vi "Power ON-Single.vi"(8 "error in":errorcluster, 11 "Power ON single":T1={"Voltage/current level"=0.0, "Voltage/current limit"=0.0, "Sense"=1009, "Resource name"="", "Output function"=1006} {"Output function" items=["DC Voltage"=1006, "DC Current"=1007, "Pulse Voltage"=1049, "Pulse Current"=1050]; "Sense" items=["Local"=1008, "Remote"=1009]}) -> (0 "error out":errorcluster, 3 "Status":string)   [LabVIEW 2021]
doc: "This VI will configure the source device to DC Current or DC Voltage mode to ower on the DUT for single channel configuration."
uses:
  controls/Power ON-Single.ctl
  <instrlib>/niDCPower/nidcpower.llb/niDCPower Source Mode.ctl
  <instrlib>/niDCPower/nidcpower.llb/niDCPower Wait For Event - Event.ctl
  <instrlib>/niDCPower/nidcpower.llb/niDCPower Get Channel Name From String.vi
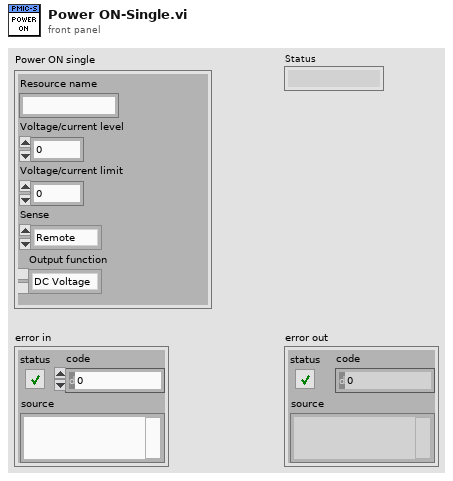
[diagram p1: front panel]
types:
  T1 = typedef "Power ON-Single.ctl" = cluster{"Voltage/current level":dbl, "Voltage/current limit":dbl, "Sense":i32, "Resource name":string, "Output function":i32}
  T2 = typedef "niDCPower Wait For Event - Event.ctl" = i32
  T3 = typedef "niDCPower Source Mode.ctl" = i32
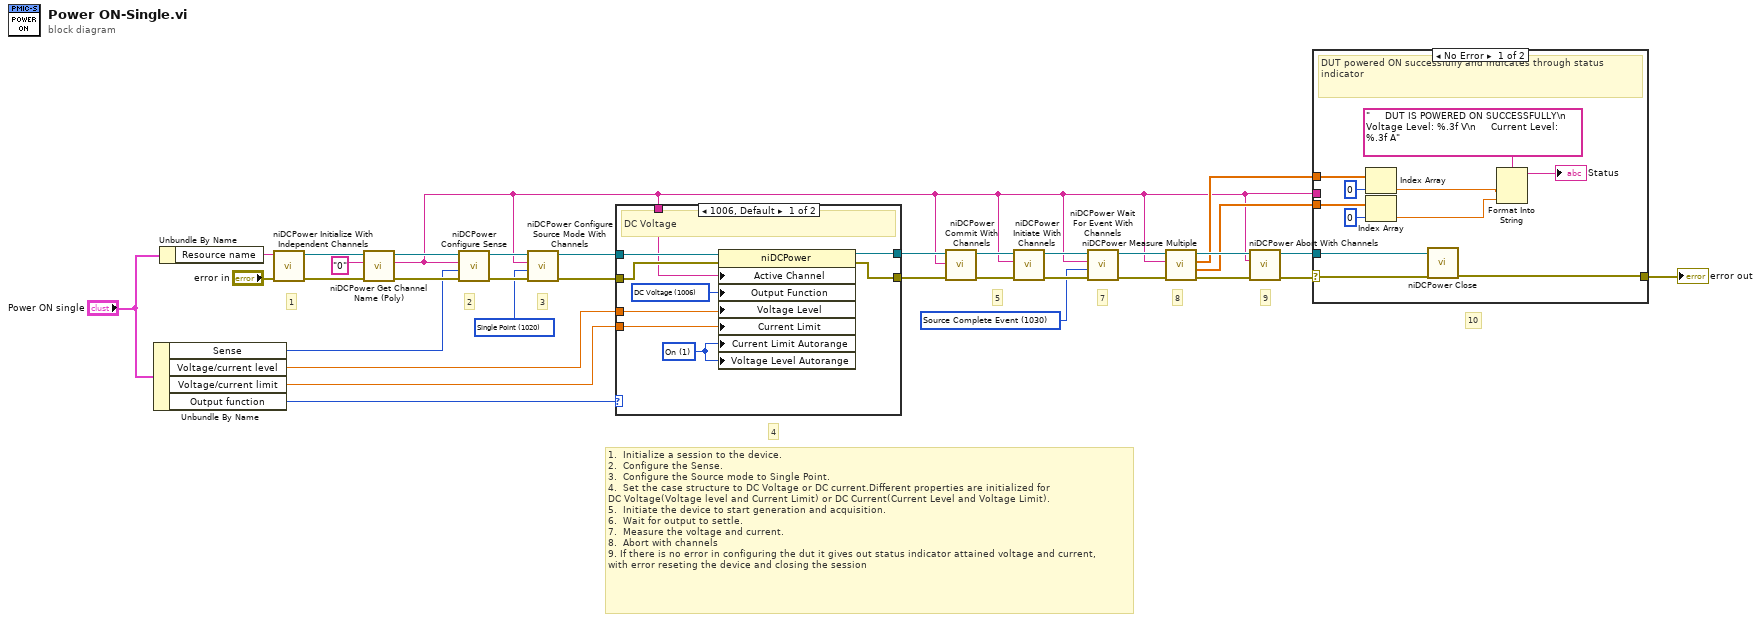
[diagram p0: block diagram]
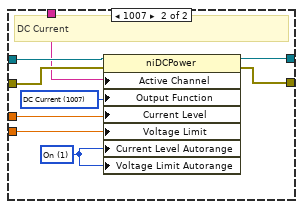
[diagram p2: hidden frame]
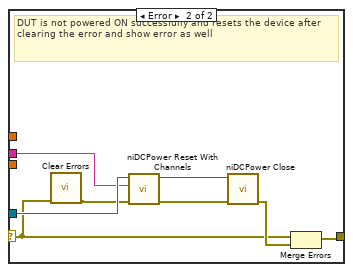
[diagram p3: hidden frame]
diagram:
  w22 = T2 1030 items=["Source Complete Event"=1030, "Measure Complete Event"=1031, "Sequence Iteration Complete Event"=1032, "Sequence Engine Done Event"=1033, "Pulse Complete Event"=1051, "Ready For Pulse Trigger Event"=1052] ("event")
  w27 = T3 1020 items=["Single Point"=1020, "Sequence"=1021] ("source mode")
  # "10"
  # "9"
  # "8"
  # "7"
  # "5"
  # "4"
  # "3"
  # "2"
  # "1"
  # "1.  Initialize a session to the device.\n2.  Configure the Sense.\n3.  Configure the Source mode to Single Point.\n4.  Set the case structure to DC Voltage or DC current.Different properties are initialized for \nDC Voltage(Voltage level and Current Limit) or DC Current(Current Level and Voltage Limit). \n5.  Initiate the device to start generation and acquisition.\n6.  Wait for output to settle.\n7.  Measure the voltage and current.\n8.  Abort with channels\n9. If there is no error in configuring the dut it gives out status indicator attained voltage and current,\nwith error reseting the device and closing the session"
  n1 = Unbundle By Name("Power ON single") -> ("Sense"=w1:i32, "Voltage/current level"=w7:dbl, "Voltage/current limit"=w6:dbl, "Output function"=w5:i32)
  n2 = Unbundle By Name("Power ON single") -> ("Resource name"=w13:string)
  n3 = call <instrlib>:"niDCPower Initialize With Independent Channels.vi"("error in (no error)"="error in", "resource name"=w13) -> ("error out"=w34:errorcluster, "instrument handle out"=w33:refnum<k15>)  [unwired: 8 in]
  n4 = call-poly <instrlib>:"niDCPower Get Channel Name (Poly).vi"("error in (no error)"=w34, "index"="0", "instrument handle"=w33) -> ("error out"=w31:errorcluster, "name"=w8:string, "instrument handle out"=w30:refnum<k15>)  [unwired: 6 in]
  n5 = call <instrlib>:"niDCPower Configure Sense.vi"("error in (no error)"=w31, "sense"=w1, "channel name"=w8, "instrument handle"=w30) -> ("error out"=w29:errorcluster, "instrument handle out"=w28:refnum<k15>)  [unwired: 6 in]
  n6 = call <instrlib>:"niDCPower Configure Source Mode With Channels.vi"("error in (no error)"=w29, "source mode"=w27, "channel name"=w8, "instrument handle"=w28) -> ("error out"=w11:errorcluster, "instrument handle out"=w12:refnum<k15>)  [unwired: 6 in]
  n7 = case shown="1006, Default" w5 {
    tunnel: w12 -> [w42 w48]
    tunnel: w11 -> [w41 w47]
    tunnel: [w40 w50] -> w10
    tunnel: [w39 w49] -> w9
    tunnel: w8 -> [w38 w46]
    tunnel: w7 -> [w37 w45]
    tunnel: w6 -> [w35 w44]
    frame 1006, Default {
      w36 = 1 items=["Off", "On"] ("Source:DC Voltage:Current Limit Autorange")
      w43 = 1006 items=["DC Voltage"=1006, "DC Current"=1007, "Pulse Voltage"=1049, "Pulse Current"=1050] ("Source:Output Function")
      # "DC Voltage"
      n8 = property class="niDCPower"(reference=w42, error in=w41, "Active Channel"=w38, "Output Function"=w43, "Voltage Level"=w37, "Current Limit"=w35, "Current Limit Autorange"=w36, "Voltage Level Autorange"=w36) -> (reference out=w40:refnum<k15>, error out=w39:errorcluster)
    }
    frame 1007 {
      w51 = 1 items=["Off", "On"] ("Source:DC Voltage:Voltage Level Autorange")
      w52 = 1007 items=["DC Voltage"=1006, "DC Current"=1007, "Pulse Voltage"=1049, "Pulse Current"=1050] ("Source:Output Function")
      # "DC Current"
      n9 = property class="niDCPower"(reference=w48, error in=w47, "Active Channel"=w46, "Output Function"=w52, "Current Level"=w45, "Voltage Limit"=w44, "Current Level Autorange"=w51, "Voltage Limit Autorange"=w51) -> (reference out=w50:refnum<k15>, error out=w49:errorcluster)
    }
  }
  n10 = call <instrlib>:"niDCPower Commit With Channels.vi"("error in (no error)"=w9, "channel name"=w8, "instrument handle"=w10) -> ("error out"=w25:errorcluster, "instrument handle out"=w26:refnum<k15>)  [unwired: 7 in]
  n11 = call <instrlib>:"niDCPower Initiate With Channels.vi"("error in (no error)"=w25, "channel name"=w8, "instrument handle"=w26) -> ("error out"=w23:errorcluster, "instrument handle out"=w24:refnum<k15>)  [unwired: 7 in]
  n12 = call <instrlib>:"niDCPower Wait For Event With Channels.vi"("error in (no error)"=w23, "event"=w22, "channel name"=w8, "instrument handle"=w24) -> ("error out"=w21:errorcluster, "instrument handle out"=w20:refnum<k15>)  [unwired: 6 in]
  n13 = call <instrlib>:"niDCPower Measure Multiple.vi"("error in (no error)"=w21, "channel name"=w8, "instrument handle"=w20) -> ("error out"=w19:errorcluster, "current measurements"=w14:dbl[], "voltage measurements"=w15:dbl[], "instrument handle out"=w18:refnum<k15>)  [unwired: 5 in]
  n14 = call <instrlib>:"niDCPower Abort With Channels.vi"("error in (no error)"=w19, "channel name"=w8, "instrument handle"=w18) -> ("error out"=w17:errorcluster, "instrument handle out"=w16:refnum<k15>)  [unwired: 7 in]
  n15 = case shown="No Error" w17 {
    selector: w17 -> [w63 w65]
    tunnel: w16 -> [w62 w71]
    tunnel: w15 -> [w61 _]
    tunnel: w14 -> [w60 _]
    tunnel: w8 -> [_ w70]
    tunnel: [w54 w64] -> w2
    frame No Error {
      # "DUT powered ON successfully and indicates through status indicator"
      n16 = Index Array(array=w61, index=0) -> (element=w57:dbl)
      n17 = Index Array(array=w60, index=0) -> (element=w56:dbl)
      n18 = call <instrlib>:"niDCPower Close.vi"("error in (no error)"=w63, "instrument handle"=w62) -> ("error out"=w54:errorcluster)  [unwired: 9 in]
      n19 = Format Into String(format string="     DUT IS POWERED ON SUCCESSFULLY\n     Voltage Level: %.3f V\n     Current Level: %.3f A", w57, w56) -> (resulting string=→"Status":string)  [unwired: 2 in, 1 out]
    }
    frame Error {
      # "DUT is not powered ON successfully and resets the device after clearing the error and show error as well"
      n20 = call <vilib>:"Clear Errors.vi"("error in (no error)"=w65) -> ("error out"=w67:errorcluster)  [unwired: 5 in, 1 out]
      n21 = call <instrlib>:"niDCPower Reset With Channels.vi"("error in (no error)"=w67, "channel name"=w70, "instrument handle"=w71) -> ("error out"=w69:errorcluster, "instrument handle out"=w68:refnum<k15>)  [unwired: 7 in]
      n22 = call <instrlib>:"niDCPower Close.vi"("error in (no error)"=w69, "instrument handle"=w68) -> ("error out"=w66:errorcluster)  [unwired: 9 in]
      n23 = Merge Errors(w65, w66) -> (w64:errorcluster)
    }
  }
  "error out" <- w2
